vi "Get Parameters in Word.vi"(8 "error in":errorcluster, 11 "word ref":T1 format="%.0x") -> (0 "error out":errorcluster, 1 "parameter definitions":T2[](array[typedef]), 2 "parameter refs":T1[](array[typedef]) format="%.0x", 3 "word ref out":T1 format="%.0x")   [LabVIEW 2020, in "ARINC 429 Scripting.lvlib"]
uses:
  ARINC 429 Scripting.lvlib
  <vilib>/NI VeriStand/Custom Device API/Custom Device Item Ref.ctl
  Shared/Parameter Definition.ctl
  <vilib>/addons/VeriStand Custom Device Scripting APIs/Ballard ARINC 429/Encoding and Decoding/Encoding.ctl
  <vilib>/NI VeriStand/Custom Device API/Custom Device API.lvlib
  <vilib>/addons/VeriStand Custom Device Scripting APIs/Ballard ARINC 429/Encoding and Decoding/Encoding and Decoding.lvlib
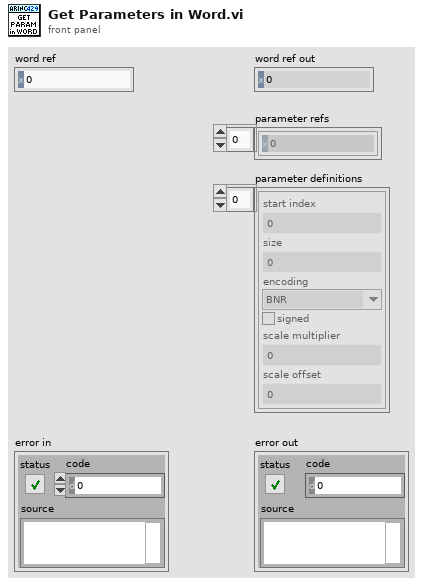
[diagram p1: front panel]
types:
  T1 = typedef "Custom Device API.lvlib/Custom Device Item Ref.ctl" = u64
  T2 = typedef "Parameter Definition.ctl" = cluster{"start index":i32, "size":i32, "encoding":T3, "signed":bool, "scale multiplier":dbl, "scale offset":dbl}
  T3 = typedef "Encoding and Decoding.lvlib/Encoding.ctl" = enum16{"BNR", "BCD", "Discrete"}
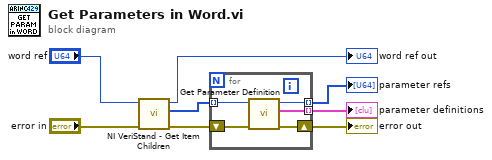
[diagram p0: block diagram]
diagram:
  n1 = call <vilib>:"NI VeriStand - Get Item Children.vi"("error in (no error)"="error in", "Item Ref in"="word ref") -> ("error out"=w2:errorcluster, "Child Refs"=w4:T1[], "Item Ref out"=→"word ref out":T1)  [unwired: 6 in, 1 out]
  n2 = for {
    shift-right: [w12] -> w3
    shift-left: w2 -> [w13]
    tunnel: w4 -> [w11] mode=indexing
    tunnel: [w10] -> w5 mode=indexing
    tunnel: [w9] -> w6 mode=indexing
    n3 = call "Get Parameter Definition.vi"("error in"=w13, "parameter ref in"=w11) -> ("error out"=w12:errorcluster, "parameter definition"=w10:T2, "parameter ref out"=w9:T1)  [unwired: 7 in]
  }
  "parameter refs" <- w6
  "parameter definitions" <- w5
  "error out" <- w3
